vi "Thermal Camera 2.vi"() -> ()   [LabVIEW 2024]
uses:
  irDirectSDK/examples/labview/libirimager_direct_binding.lvlib
panel:
  out "height out":i32
  out "width out":i32
  in  "Connect_usb":bool
  out "Thermal Image":picture
  in  "stop":bool
  out "Successfully Connected":i32
  in  "xml_config":string
  out "function return 2":i32
  out "thermal data out":u16[](array[numeric])
  out "function return":i32
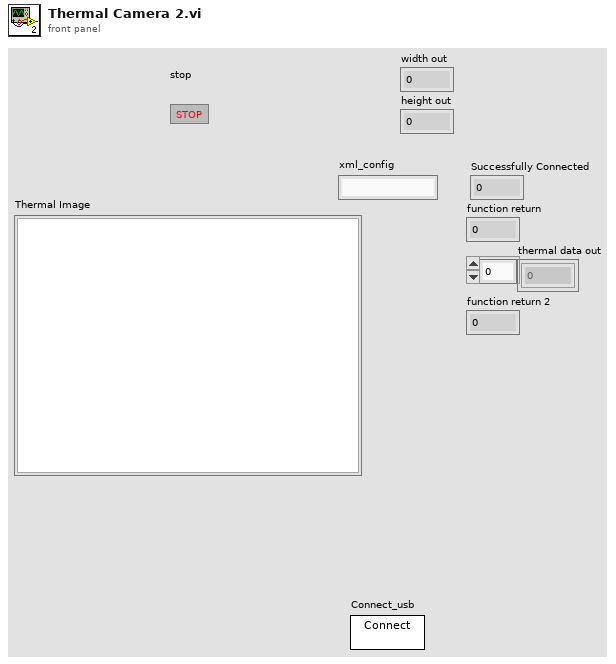
[diagram p1: front panel]
types:
  T1 = typedef "imagedata.ctl" = cluster{"image type":i32, "image depth":i32, "image":u8[], "mask":u8[], "colors":u32[], "Rectangle":cluster{"left":i16, "top":i16, "right":i16, "bottom":i16}}
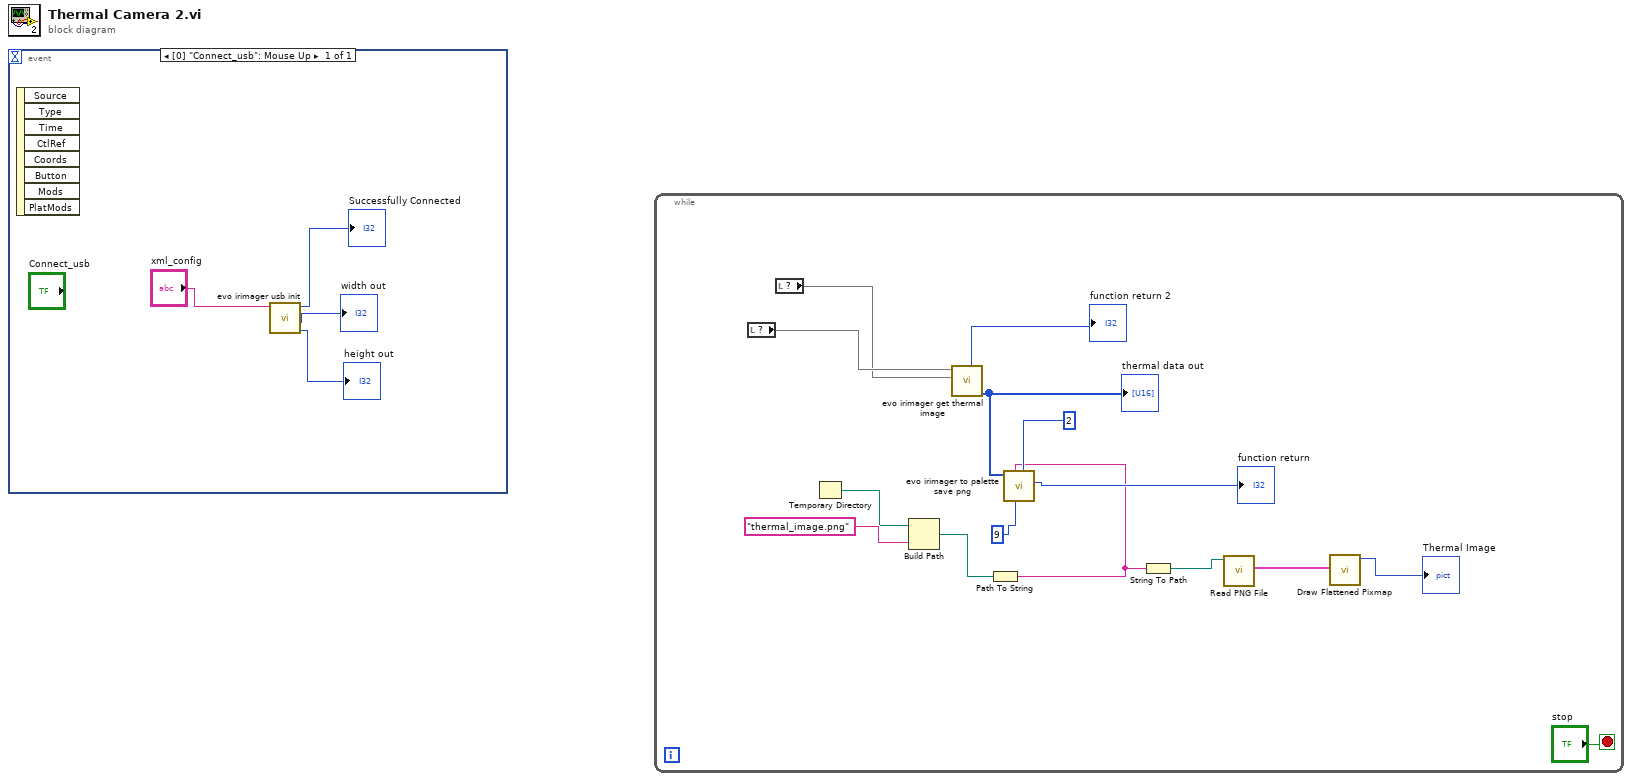
[diagram p0: block diagram]
diagram:
  n1 = event shown="[0] \"Connect_usb\": Mouse Up" {
    selector: _ -> [_]
    dyn-events: _ -> [_]
    timeout: _ -> [_]
    event "Connect_usb": Mouse Up {
      n2 = event-data() -> ()  [unwired: 1 in, 8 out]
      n3 = call "evo irimager usb init.vi"("xml_config"="xml_config") -> ("h out"=→"height out":i32, "w out"=→"width out":i32, "function return 2"=→"Successfully Connected":i32)  [unwired: 7 in, 1 out]
    }
  }
  n4 = while {
    stop <- "stop" stop-if-true
    n5 = local read item#-1() -> (w6)
    n6 = local read item#-1() -> (w5)
    n7 = Temporary Directory() -> (w12:path)
    n8 = Build Path(base path=w12, name or relative path="thermal_image.png") -> (appended path=w14:path)
    n9 = call "evo irimager get thermal image.vi"("h"=w5, "w"=w6) -> ("data out"=w16:u16[], "function return"=→"function return 2":i32)  [unwired: 6 in, 2 out]
    "thermal data out" <- w16
    n10 = Path To String(path=w14) -> (string=w11:string)
    n11 = call "evo irimager to palette save png.vi"("palette_scale"=2, "palette"=9, "path"=w11, "thermal_data"=w16) -> ("function return"=→"function return":i32)  [unwired: 6 in, 1 out]
    n12 = String To Path(string=w11) -> (path=w10:path)
    n13 = call <vilib>:"Read PNG File.vi"("path to PNG file"=w10) -> ("image data"=w8:T1)  [unwired: 8 in, 2 out]
    n14 = call <vilib>:"Draw Flattened Pixmap.vi"("image data"=w8) -> ("new picture"=→"Thermal Image":picture)  [unwired: 8 in]
  }
